vi "Parse-Is_White.vi"(10 "Color":u32(colorbox)=16777215) -> (1 "Color Cluster":T2={"R"=255, "G"=255, "B"=255, "Color Box"=16777215}, 2 "Is White":bool=TRUE, 3 "Tile Color":T1)   [LabVIEW 2020]
doc: "<B>Description:</B> Takes a color and determines if it is close enough to white to be considered traversable for maze purposes.\n\n<B>Date:</B> 1/2019\n<B>Author:</B> Luke Jarocki, Choose Movement Consulting, LLC"
uses:
  Controls/Split_Color.ctl
  Controls/TileColor.ctl
panel:
  in  "White Threshold":u8=80
  out "R":u8=255 format="%.0x"
  out "G":u8=255 format="%.0x"
  out "B":u8=255 format="%.0x"
  # "Is White?"
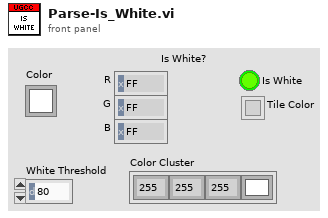
[diagram p1: front panel]
types:
  T1 = typedef "TileColor.ctl" = u16
  T2 = typedef "Split_Color.ctl" = cluster{"R":u8, "G":u8, "B":u8, "Color Box":u32}
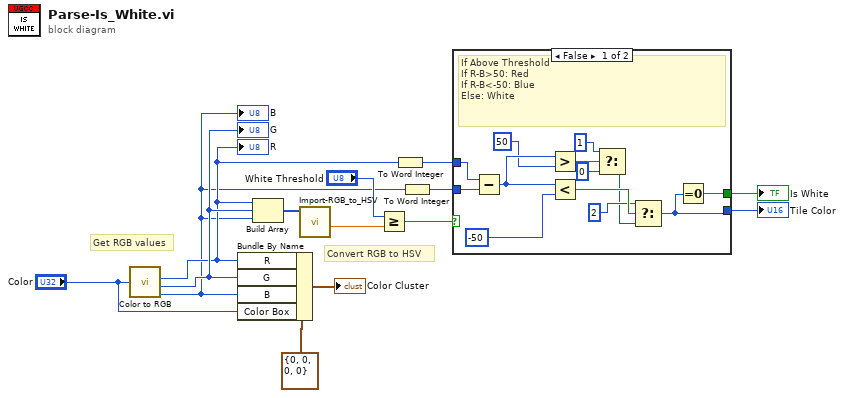
[diagram p0: block diagram]
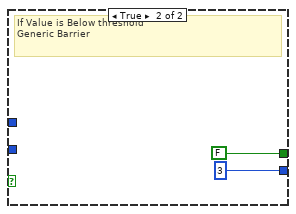
[diagram p2: hidden frame]
diagram:
  # "Convert RGB to HSV"
  # "Get RGB values"
  n1 = call <vilib>:"Color to RGB.vi"("Color"="Color") -> ("R"=w4:u8, "G"=w11:u8, "B"=w3:u8)  [unwired: 1 out]
  "B" <- w3
  "G" <- w11
  "R" <- w4
  n2 = Bundle By Name(cluster=T2 {"R"=0, "G"=0, "B"=0, "Color Box"=0} ("Cluster"), "R"=w4, "G"=w11, "B"=w3, "Color Box"="Color") -> (→"Color Cluster":T2)
  n3 = Build Array(w4, w11, w3) -> (w10:u8[])
  n4 = call "Import-RGB_to_HSV.vi"("RGB"=w10) -> ("Value"=w9:dbl)  [unwired: 7 in, 3 out]
  n5 = Greater Or Equal?(x="White Threshold", y=w9) -> (x >= y?=w7:bool)
  n6 = To Word Integer(number=w4) -> (16bit integer=w2:i16)
  n7 = To Word Integer(number=w3) -> (16bit integer=w1:i16)
  n8 = case shown="False" w7 {
    tunnel: [w15 FALSE] -> w6
    tunnel: [w16 T1 3 ("Is white")] -> w5
    tunnel: w2 -> [w27 _]
    tunnel: w1 -> [w26 _]
    frame False {
      # "If Above Threshold\nIf R-B>50: Red\nIf R-B<-50: Blue\nElse: White"
      n9 = Subtract(x=w27, y=w26) -> (x-y=w24:i16)
      n10 = Greater?(x=w24, y=i16 50 ("x")) -> (0:w22:bool)
      n11 = Less?(x=w24, y=i16 -50 ("x")) -> (x < y?=w19:bool)
      n12 = Select(t=T1 1 ("Is white"), s=w22, f=T1 0 ("Is white")) -> (s? t:f=w17:T1)
      n13 = Select(t=T1 2 ("Is white"), s=w19, f=w17) -> (s? t:f=w16:T1)
      n14 = Equal To 0?(x=w16) -> (x = 0?=w15:bool)
    }
    frame True {
      # "If Value is Below threshold\nGeneric Barrier"
    }
  }
  "Is White" <- w6
  "Tile Color" <- w5
